vi "Write Calibration 1.vi"(8 "error in (no error)":errorcluster, 10 "RP EEPROM Calibration":T1 {"magic" format="%x"}, 11 "RP Instrument in":refnum<class "RP Instrument.lvclass">) -> (0 "error out":errorcluster, 3 "RP Instrument out":refnum<class "RP Instrument.lvclass">)   [LabVIEW 2019, in "RP Instrument.lvclass"]
uses:
  RP Instrument.lvclass
  RP EEPROM Calibration.ctl
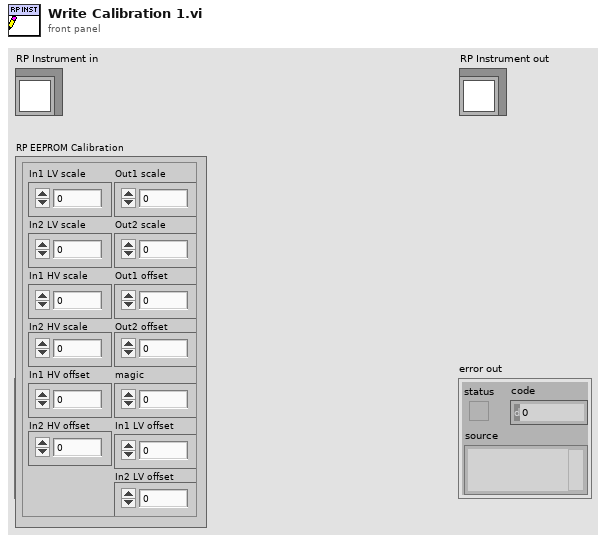
[diagram p1: front panel]
types:
  T1 = typedef "RP EEPROM Calibration.ctl" = cluster{"In1 LV scale":u32, "In2 LV scale":u32, "In1 HV scale":u32, "In2 HV scale":u32, "In1 HV offset":i32, "In2 HV offset":i32, "Out1 scale":u32, "Out2 scale":u32, "Out1 offset":i32, "Out2 offset":i32, "magic":u32, "In1 LV offset":i32, "In2 LV offset":i32}
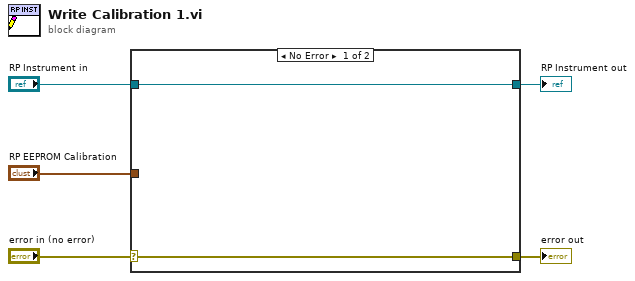
[diagram p0: block diagram]
diagram:
  n1 = case shown="No Error" "error in (no error)" {
    selector: "error in (no error)" -> [w7 w8]
    tunnel: [w7 w8] -> w4
    tunnel: [w6 w9] -> w2
    tunnel: "RP Instrument in" -> [w6 w9]
    tunnel: "RP EEPROM Calibration" -> [_ _]
    frame No Error {
    }
    frame Error {
    }
  }
  "error out" <- w4
  "RP Instrument out" <- w2
